vi "3.1.vi"() -> ()   [LabVIEW 2017]
panel:
  out "余弦":dbl
  out "正弦":dbl
  in  "输入":dbl
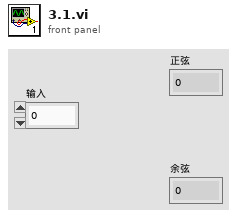
[diagram p1: front panel]
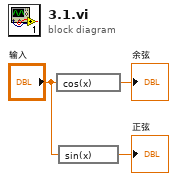
[diagram p0: block diagram]
diagram:
  n1 = expression code="cos(x)"("输入") -> (→"余弦":dbl)
  n2 = expression code="sin(x)"("输入") -> (→"正弦":dbl)
